vi "Read Refnum Groups.vi"(11 "All Controls in":T1) -> (0 "Not Boolean":refnum<vi>[](array[refnum]), 1 "Switching Boolean":refnum<vi>[](array[refnum]), 2 "Latching Boolean":refnum<vi>[](array[refnum]), 3 "All Controls":refnum<vi>[](array[refnum]))   [LabVIEW 2017, in "AutoRegistration.lvlib" / "AutoRegistration.lvclass"]
doc: "<License>\nCopyright © 2017 Composed Systems, LLC | All rights reserved\nwww.composed.io\n\nAuthor: Ethan Stern <ethan.stern@composed.io>\n\nThis software is provided \"AS IS\" WITHOUT WARRANTIES, either express or implied, AND IS FOR EDUCATIONAL PURPOSES ONLY.\n</License>"
uses:
  AutoRegistration.lvclass
  Registration References.ctl
panel:
  # "This subVI assigns owned labels\nto the auto-registered references"
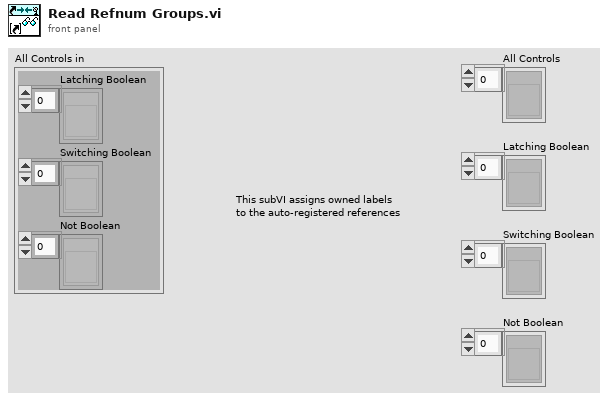
[diagram p1: front panel]
types:
  T1 = typedef "AutoRegistration.lvlib/AutoRegistration.lvclass/Registration References.ctl" = cluster{"Latching Boolean":refnum<vi>[], "Switching Boolean":refnum<vi>[], "Not Boolean":refnum<vi>[]}
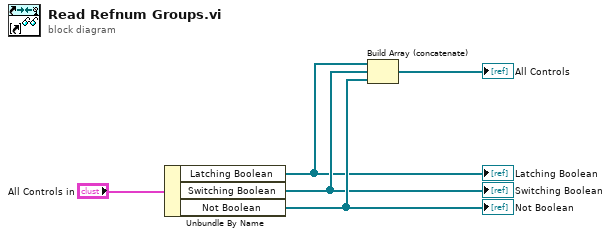
[diagram p0: block diagram]
diagram:
  n1 = Unbundle By Name("All Controls in") -> ("Latching Boolean"=w2:refnum<vi>[], "Switching Boolean"=w3:refnum<vi>[], "Not Boolean"=w4:refnum<vi>[])
  "Not Boolean" <- w4
  "Switching Boolean" <- w3
  "Latching Boolean" <- w2
  n2 = Build Array (concatenate)(w2, w3, w4) -> (→"All Controls":refnum<vi>[])
